vi "Safe_Serial_tl.vi"(1 "Tx String":string, 3 "Terminator (glob)":string, 4 "Echo Checking (F)":bool, 5 "Timeout Checking (T)":bool=TRUE, 6 "Serial Error Check (T)":bool=TRUE, 7 "Timeout (glob)":dbl=nan format="%.2f") -> (0 "Rx String":string, 2 "TxRx OK?":bool)   [LabVIEW 2010]
doc: "This VI repeatedly uses the serial communication VI until it succesfully receives a reply."
uses:
  Serial_Setup_tl.glob.vi
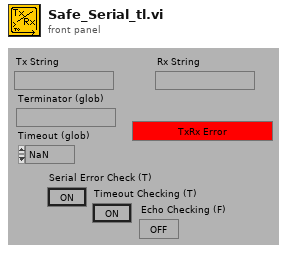
[diagram p1: front panel]
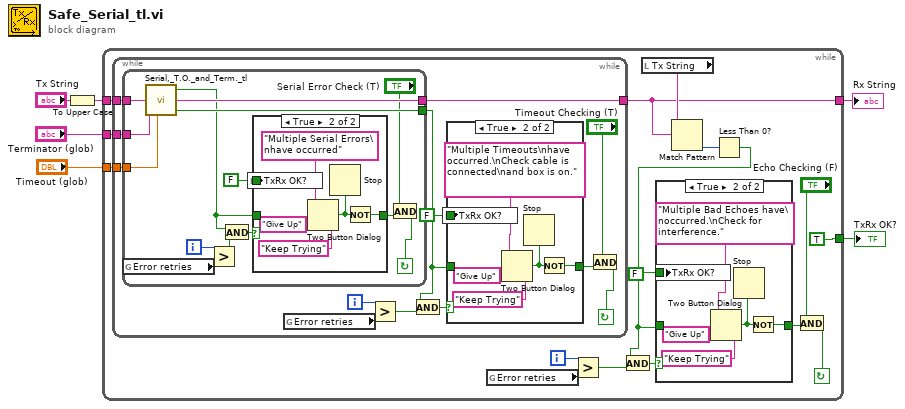
[diagram p0: block diagram]
diagram:
  n1 = To Upper Case(1:"Tx String") -> (0:w4:string)
  n2 = while {
    tunnel: [TRUE] -> w1
    tunnel: "Terminator (glob)" -> [w9]
    tunnel: "Timeout (glob)" -> [w10]
    tunnel: [w14] -> w5
    tunnel: w4 -> [w18]
    i -> [w22]
    stop <- w19 continue-if-true
    n3 = while {
      tunnel: w9 -> [w24]
      tunnel: w10 -> [w25]
      tunnel: w18 -> [w30]
      tunnel: [w31] -> w14
      i -> [w35]
      stop <- w32 continue-if-true
      n4 = while {
        tunnel: w24 -> [w37]
        tunnel: w25 -> [w38]
        tunnel: w30 -> [w45]
        tunnel: [w46] -> w31
        tunnel: [w47] -> w28
        i -> [w49]
        stop <- w40 continue-if-true
        n5 = global read "Serial_Setup_tl.glob.vi" "Error retries"() -> (w48:i32)
        n6 = call "Serial,_T.O._and_Term._tl.vi"("Write String"=w45, "Terminator"=w37, "Timeout"=w38) -> ("Serial Error"=w42:bool, "Read"=w46:string, "T.O."=w47:bool)  [unwired: 4 out]
        n7 = Greater?(x=w49, y=w48) -> (0:w43:bool)
        n8 = And(x=w42, y=w43) -> (x .and. y?=w44:bool)
        n9 = case shown="True" w44 {
          tunnel: w42 -> [w50 _]
          tunnel: [w50 w52] -> w41
          tunnel: FALSE -> [_ w51]
          frame False {
          }
          frame True {
            n10 = local write "TxRx OK?"(w51) -> ()
            n11 = Two Button Dialog(message="Multiple Serial Errors\nhave occurred", 1:"Keep Trying", 2:"Give Up") -> (T button?=w53:bool)
            n12 = Stop(stop? (T)=w53) -> ()
            n13 = Not(x=w53) -> (.not. x?=w52:bool)
          }
        }
        n14 = And(x="Serial Error Check (T)", y=w41) -> (x .and. y?=w40:bool)
      }
      n15 = global read "Serial_Setup_tl.glob.vi" "Error retries"() -> (w34:i32)
      n16 = Greater?(x=w35, y=w34) -> (0:w27:bool)
      n17 = And(x=w28, y=w27) -> (x .and. y?=w26:bool)
      n18 = case shown="True" w26 {
        tunnel: w28 -> [w57 _]
        tunnel: [w57 w59] -> w33
        tunnel: FALSE -> [_ w58]
        frame False {
        }
        frame True {
          n19 = local write "TxRx OK?"(w58) -> ()
          n20 = Two Button Dialog(message="Multiple Timeouts\nhave occurred.\nCheck cable is connected\nand box is on.", 1:"Keep Trying", 2:"Give Up") -> (T button?=w60:bool)
          n21 = Stop(stop? (T)=w60) -> ()
          n22 = Not(x=w60) -> (.not. x?=w59:bool)
        }
      }
      n23 = And(x="Timeout Checking (T)", y=w33) -> (x .and. y?=w32:bool)
    }
    n24 = global read "Serial_Setup_tl.glob.vi" "Error retries"() -> (w21:i32)
    n25 = Greater?(x=w22, y=w21) -> (0:w12:bool)
    n26 = local read "Tx String"() -> (w17:string)
    n27 = Match Pattern(string=w14, regular expression=w17) -> (offset past match=w15:i32)  [unwired: 4 out]
    n28 = Less Than 0?(x=w15) -> (x < 0?=w13:bool)
    n29 = And(x=w13, y=w12) -> (x .and. y?=w11:bool)
    n30 = case shown="True" w11 {
      tunnel: w13 -> [w64 _]
      tunnel: [w64 w65] -> w20
      tunnel: FALSE -> [_ w66]
      frame False {
      }
      frame True {
        n31 = local write "TxRx OK?"(w66) -> ()
        n32 = Two Button Dialog(message="Multiple Bad Echoes have\noccurred.\nCheck for interference.", 1:"Keep Trying", 2:"Give Up") -> (T button?=w67:bool)
        n33 = Stop(stop? (T)=w67) -> ()
        n34 = Not(x=w67) -> (.not. x?=w65:bool)
      }
    }
    n35 = And(x="Echo Checking (F)", y=w20) -> (x .and. y?=w19:bool)
  }
  "Rx String" <- w5
  "TxRx OK?" <- w1
